vi "Read and Write Cards.vi"(8 "error in (no error)":errorcluster, 11 "PXI in":refnum<class "PXI.lvclass">) -> (0 "error out":errorcluster, 3 "PXI out":refnum<class "PXI.lvclass">)   [LabVIEW 2013, in "PXI.lvclass"]
uses:
  PXI.lvclass
  PXI.lvclass/PXI.ctl
  <vilib>/DAQmx/read.llb/DAQmx Read (Analog 1D DBL NChan 1Samp).vi
  <vilib>/DAQmx/write.llb/DAQmx Write (Analog 1D DBL NChan 1Samp).vi
  <vilib>/DAQmx/read.llb/DAQmx Read (Digital 1D Bool NChan 1Samp 1Line).vi
  <vilib>/DAQmx/write.llb/DAQmx Write (Digital 1D Bool NChan 1Samp 1Line).vi
  <vilib>/DAQmx/miscellaneous.llb/DAQmx Fill In Error Info.vi
  <resource>/objmgr/daqmx.rc
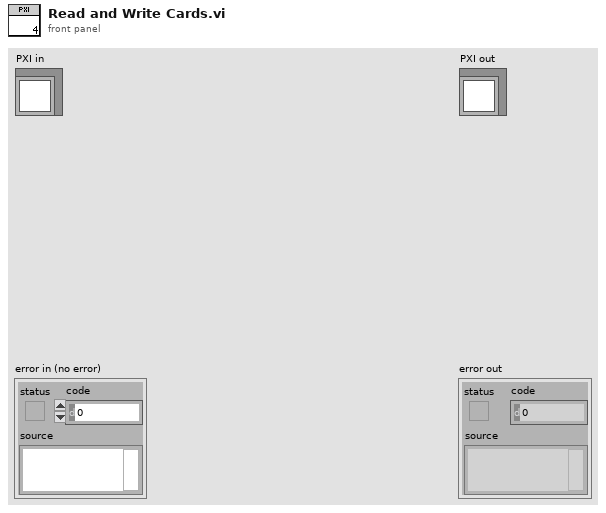
[diagram p1: front panel]
types:
  T1 = typedef "PXI.lvclass/Task Definition.ctl" = cluster{"task_type":T2, "names":string[], "physical channels":tag, "min_value":dbl, "max_value":dbl, "task_number":i32}
  T2 = typedef "PXI.lvclass/Task Types.ctl" = enum16{"Analog Input", "Analog Output", "Digital Input", "Digital Output"}
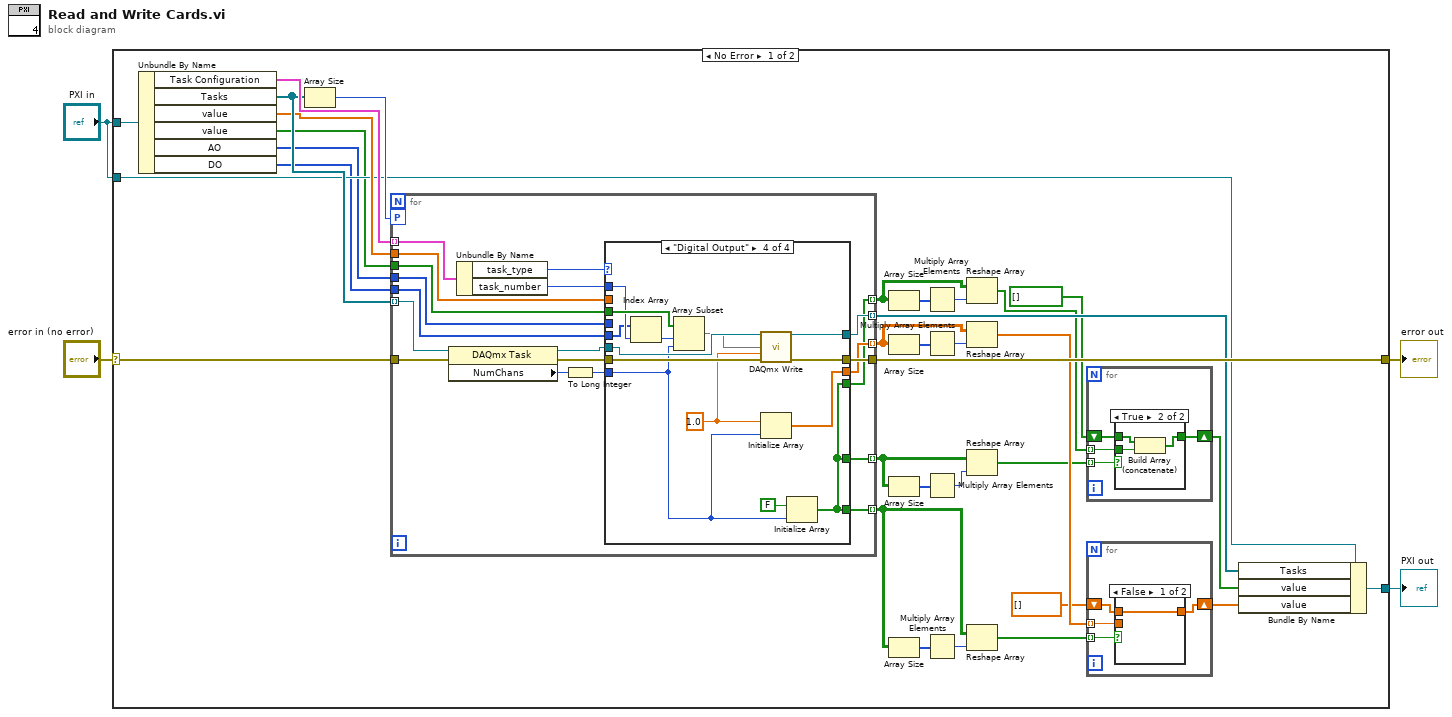
[diagram p0: block diagram]
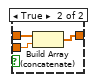
[diagram p2: hidden frame]
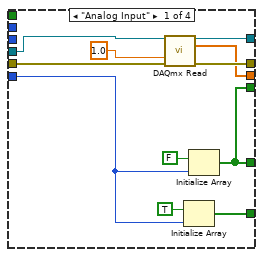
[diagram p4: hidden frame]
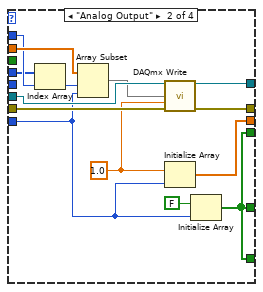
[diagram p5: hidden frame]
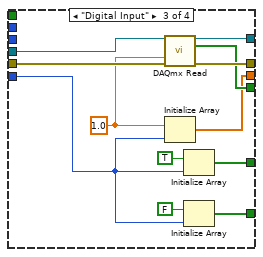
[diagram p6: hidden frame]
diagram:
  n1 = case shown="No Error" "error in (no error)" {
    selector: "error in (no error)" -> [w34 w125]
    tunnel: [w33 w125] -> w3
    tunnel: [w31 w124] -> w2
    tunnel: "PXI in" -> [w32 w124]
    tunnel: "PXI in" -> [w28 _]
    frame No Error {
      n2 = Unbundle By Name(w32) -> ("Task Configuration"=w37:T1[], "Tasks"=w36:refnum<k21>[], "value"=w29:dbl[], "value"=w21:bool[], "AO"=w20:i32[], "DO"=w19:i32[])
      n3 = Array Size(array=w36) -> (size(s)=w35:i32)
      n4 = for {
        tunnel: w37 -> [w72] mode=indexing
        tunnel: w36 -> [w68] mode=indexing
        workers-P: w35 -> [_]
        tunnel: [w69] -> w30 mode=indexing
        tunnel: w34 -> [w65]
        tunnel: [w70] -> w33
        tunnel: w29 -> [w63]
        tunnel: w21 -> [w61]
        tunnel: [w60] -> w24 mode=indexing
        tunnel: [w59] -> w27 mode=indexing
        tunnel: w20 -> [w57]
        tunnel: w19 -> [w56]
        tunnel: [w55] -> w10 mode=indexing
        tunnel: [w54] -> w13 mode=indexing
        n5 = property class="DAQmx Task"(reference=w68, error in=w65) -> (reference out=w67:refnum<k21>, error out=w66:errorcluster, "NumChans"=w64:u32)
        n6 = Unbundle By Name(w72) -> ("task_type"=w71:T2, "task_number"=w58:i32)
        n7 = To Long Integer(number=w64) -> (32bit integer=w62:i32)
        n8 = case shown="\"Digital Output\"" w71 {
          tunnel: w67 -> [w82 w97 w109 w123]
          tunnel: w66 -> [w80 w96 w107 w121]
          tunnel: [w81 w95 w108 w122] -> w70
          tunnel: [w79 w94 w106 w120] -> w69
          tunnel: w63 -> [_ w92 _ _]
          tunnel: w62 -> [w75 w86 w99 w111]
          tunnel: w61 -> [_ _ _ w119]
          tunnel: [w78 w85 w98 w112] -> w60
          tunnel: [w73 w84 w105 w110] -> w59
          tunnel: w58 -> [_ w91 _ w117]
          tunnel: w57 -> [_ w90 _ _]
          tunnel: w56 -> [_ _ _ w116]
          tunnel: [w73 w84 w103 w110] -> w55
          tunnel: [w77 w84 w102 w110] -> w54
          frame "Analog Input" {
            n9 = call-poly <vilib>:"DAQmx Read.vi"("task/channels in"=w82, "timeout"=1.0, "error in"=w80) -> ("task out"=w79:refnum<k21>, "data"=w78:dbl[], "error out"=w81:errorcluster)  [unwired: 10 in]
            n10 = Initialize Array(TRUE, w75) -> (w77:bool[])
            n11 = Initialize Array(FALSE, w75) -> (w73:bool[])
          }
          frame "Analog Output" {
            w87 = 1.0 ("data")
            n12 = Index Array(array=w90, index=w91) -> (element=w89:i32)
            n13 = Array Subset(array=w92, index=w89, length=w86) -> (w93:dbl[])
            n14 = call-poly <vilib>:"DAQmx Write.vi"("task/channels in"=w97, "data"=w93, "timeout"=w87, "error in"=w96) -> ("task out"=w94:refnum<k21>, "error out"=w95:errorcluster)  [unwired: 9 in, 1 out]
            n15 = Initialize Array(w87, w86) -> (w85:dbl[])
            n16 = Initialize Array(FALSE, w86) -> (w84:bool[])
          }
          frame "Digital Input" {
            w100 = 1.0 ("timeout")
            n17 = call-poly <vilib>:"DAQmx Read.vi"("task/channels in"=w109, "timeout"=w100, "error in"=w107) -> ("task out"=w106:refnum<k21>, "data"=w105:bool[], "error out"=w108:errorcluster)  [unwired: 10 in]
            n18 = Initialize Array(w100, w99) -> (w98:dbl[])
            n19 = Initialize Array(TRUE, w99) -> (w103:bool[])
            n20 = Initialize Array(FALSE, w99) -> (w102:bool[])
          }
          frame "Digital Output" {
            w113 = 1.0 ("timeout")
            n21 = Index Array(array=w116, index=w117) -> (element=w115:i32)
            n22 = Array Subset(array=w119, index=w115, length=w111) -> (w118:bool[])
            n23 = call-poly <vilib>:"DAQmx Write.vi"("task/channels in"=w123, "data"=w118, "timeout"=w113, "error in"=w121) -> ("task out"=w120:refnum<k21>, "error out"=w122:errorcluster)  [unwired: 9 in, 1 out]
            n24 = Initialize Array(w113, w111) -> (w112:dbl[])
            n25 = Initialize Array(FALSE, w111) -> (w110:bool[])
          }
        }
      }
      n26 = Array Size(array=w27) -> (size(s)=w26:i32[])
      n27 = Array Size(array=w24) -> (size(s)=w23:i32[])
      n28 = Array Size(array=w10) -> (size(s)=w12:i32[])
      n29 = Array Size(array=w13) -> (size(s)=w16:i32[])
      n30 = Multiply Array Elements(1:w26) -> (0:w25:i32)
      n31 = Multiply Array Elements(1:w23) -> (0:w22:i32)
      n32 = Multiply Array Elements(1:w12) -> (0:w11:i32)
      n33 = Multiply Array Elements(1:w16) -> (0:w15:i32)
      n34 = Reshape Array(w27, w25) -> (w17:bool[])
      n35 = Reshape Array(w24, w22) -> (w18:dbl[])
      n36 = Reshape Array(w10, w11) -> (w9:bool[])
      n37 = Reshape Array(w13, w15) -> (w14:bool[])
      n38 = for {
        tunnel: w17 -> [w48] mode=indexing
        tunnel: w9 -> [w49] mode=indexing
        shift-right: [w47] -> w8
        shift-left: bool[] [] -> [w46]
        n39 = case shown="True" w49 {
          tunnel: w48 -> [_ w53]
          tunnel: [w50 w52] -> w47
          tunnel: w46 -> [w50 w51]
          frame False {
          }
          frame True {
            n40 = Build Array (concatenate)(w51, w53) -> (w52:bool[])
          }
        }
      }
      n41 = for {
        tunnel: w18 -> [w41] mode=indexing
        tunnel: w14 -> [w40] mode=indexing
        shift-right: [w39] -> w7
        shift-left: dbl[] [] -> [w38]
        n42 = case shown="False" w40 {
          tunnel: w41 -> [_ w45]
          tunnel: [w42 w44] -> w39
          tunnel: w38 -> [w42 w43]
          frame False {
          }
          frame True {
            n43 = Build Array (concatenate)(w43, w45) -> (w44:dbl[])
          }
        }
      }
      n44 = Bundle By Name(cluster=w28, "Tasks"=w30, "value"=w8, "value"=w7) -> (w31:refnum<class "PXI.lvclass">)
    }
    frame Error {
    }
  }
  "error out" <- w3
  "PXI out" <- w2
